vi "incomingEvent.vi"(8 "error in (no error)":errorcluster, 9 "data":variant, 10 "eventId":enum16{"Open", "Save", "Close"}(ring), 11 "ScriptEditorV2 in":refnum<class "ScriptEditorV2.lvclass">) -> (0 "error out":errorcluster, 1 "close":bool, 3 "ScriptEditorV2 out":refnum<class "ScriptEditorV2.lvclass">)   [LabVIEW 2011, in "Views.lvlib" / "ScriptEditor.lvlib" / "ScriptEditorV2.lvclass"]
uses:
  ScriptEditorV2.lvclass
  ScriptEditorV2.lvclass/ScriptEditorV2.ctl
  ScriptEdEvents/ScriptEdEvents.lvclass
  Tools/DatabaseHelpers.lvlib
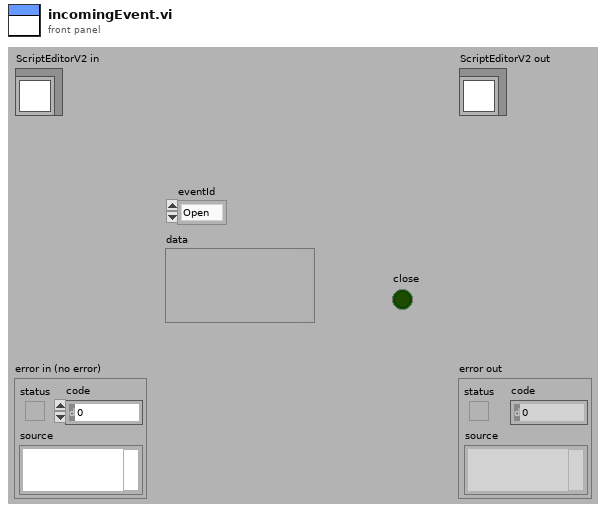
[diagram p1: front panel]
types:
  T1 = cluster{"open":cluster{"Path":path}, "close":cluster{"Boolean":bool}, "save":cluster{"Path":path}}
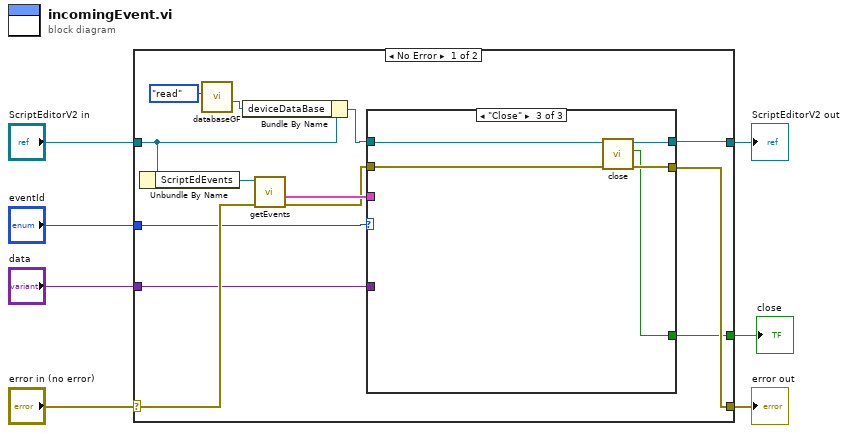
[diagram p0: block diagram]
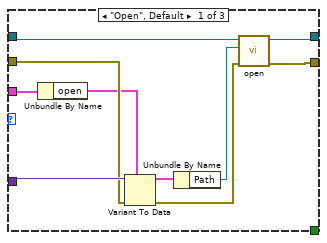
[diagram p2: hidden frame]
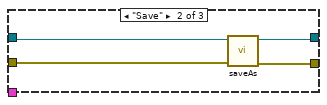
[diagram p3: hidden frame]
diagram:
  n1 = case shown="No Error" "error in (no error)" {
    selector: "error in (no error)" -> [w19 w41]
    tunnel: [w13 w41] -> w6
    tunnel: [w15 w40] -> w4
    tunnel: "ScriptEditorV2 in" -> [w10 w40]
    tunnel: "eventId" -> [w18 _]
    tunnel: "data" -> [w16 _]
    tunnel: [w12 _] -> w1
    frame No Error {
      n2 = Unbundle By Name(w10) -> ("ScriptEdEvents"=w20:refnum<class "ScriptEdEvents.lvclass">)
      n3 = call "databaseGF.vi"("Enum"=enum16{"write", "read"}."read") -> ("deviceDataBase out"=w8:refnum<class "deviceDataBase.lvclass">)  [unwired: 10 in]
      n4 = Bundle By Name(cluster=w10, "deviceDataBase"=w8) -> (w9:refnum<class "ScriptEditorV2.lvclass">)
      n5 = call-dynamic "getEvents.vi"("error in (no error)"=w19, "ScriptEdEvents in"=w20) -> ("error out"=w14:errorcluster, "eventsToScriptEd"=w17:T1)  [unwired: 6 in, 2 out]
      n6 = case shown="\"Close\"" w18 {
        tunnel: w17 -> [w30 _ _]
        tunnel: w16 -> [w27 _ _]
        tunnel: w9 -> [w29 w34 w38]
        tunnel: [w28 w33 w39] -> w15
        tunnel: w14 -> [w26 w31 w35]
        tunnel: [w21 w32 w37] -> w13
        tunnel: [_ _ w36] -> w12
        frame "Open", Default {
          n7 = Unbundle By Name(w30) -> ("open"=w25:cluster{"Path":path})
          n8 = Variant To Data(error in=w26, type=w25, Variant=w27) -> (data=w24:cluster{"Path":path}, error out=w22:errorcluster)
          n9 = Unbundle By Name(w24) -> ("Path"=w23:path)
          n10 = call "open.vi"("error in (no error)"=w22, "Path"=w23, "ScriptEditorV2 in"=w29) -> ("error out"=w21:errorcluster, "ScriptEditorV2 out"=w28:refnum<class "ScriptEditorV2.lvclass">)  [unwired: 7 in]
        }
        frame "Save" {
          n11 = call "saveAs.vi"("error in (no error)"=w31, "ScriptEditorV2 in"=w34) -> ("error out"=w32:errorcluster, "ScriptEditorV2 out"=w33:refnum<class "ScriptEditorV2.lvclass">)  [unwired: 8 in]
        }
        frame "Close" {
          n12 = call "close.vi"("error in (no error)"=w35, "ScriptEditorV2 in"=w38) -> ("error out"=w37:errorcluster, "close"=w36:bool, "ScriptEditorV2 out"=w39:refnum<class "ScriptEditorV2.lvclass">)  [unwired: 7 in]
        }
      }
    }
    frame Error {
    }
  }
  "error out" <- w6
  "ScriptEditorV2 out" <- w4
  "close" <- w1
